vi "DistPoints.vi"(10 "Point2":cluster{"X":dbl, "Y":dbl, "OnOff":bool}, 11 "Point1":cluster{"X":dbl, "Y":dbl, "OnOff":bool}) -> (3 "Distance":dbl)   [LabVIEW 2014]
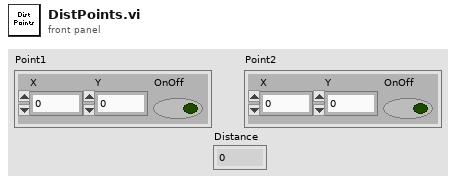
[diagram p1: front panel]
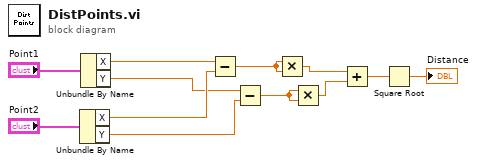
[diagram p0: block diagram]
diagram:
  n1 = Unbundle By Name("Point2") -> ("X"=w9:dbl, "Y"=w7:dbl)
  n2 = Unbundle By Name("Point1") -> ("X"=w10:dbl, "Y"=w8:dbl)
  n3 = Subtract(x=w10, y=w9) -> (x-y=w6:dbl)
  n4 = Subtract(x=w8, y=w7) -> (x-y=w5:dbl)
  n5 = Multiply(x=w6, y=w6) -> (x*y=w4:dbl)
  n6 = Multiply(x=w5, y=w5) -> (x*y=w3:dbl)
  n7 = Add(x=w4, y=w3) -> (x+y=w2:dbl)
  n8 = Square Root(x=w2) -> (sqrt(x)=→"Distance":dbl)
